vi "Open.vi"(8 "error in (no error)":errorcluster, 11 "PowerSupply-Fix in":refnum<class "PowerSupply-Fix.lvclass">) -> (0 "error out":errorcluster, 3 "PowerSupply-Fix out":refnum<class "PowerSupply-Fix.lvclass">)   [LabVIEW 2020, in "LAF2024Q2.lvlib" / "PowerSupply-Fix.lvclass"]
uses:
  PowerSupply-Fix.lvclass
  PowerSupply-Fix.lvclass/PowerSupply-Fix.ctl
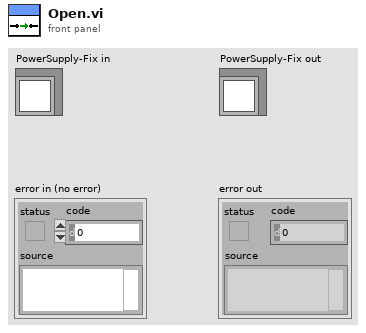
[diagram p1: front panel]
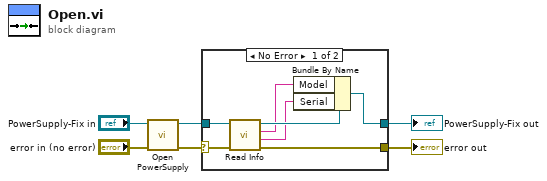
[diagram p0: block diagram]
diagram:
  n1 = call-dynamic "Open PowerSupply.vi"("error in (no error)"="error in (no error)", "PowerSupply-Fix in"="PowerSupply-Fix in") -> ("error out"=w5:errorcluster, "PowerSupply-Fix out"=w2:refnum<class "PowerSupply-Fix.lvclass">)  [unwired: 8 in]
  n2 = case shown="No Error" w5 {
    selector: w5 -> [w13 w14]
    tunnel: [w12 w14] -> w3
    tunnel: w2 -> [w11 w15]
    tunnel: [w9 w15] -> w1
    frame No Error {
      n3 = call-dynamic "Read Info.vi"("error in (no error)"=w13, "PowerSupply-Fix in"=w11) -> ("error out"=w12:errorcluster, "Serial"=w7:string, "Model"=w8:string, "PowerSupply-Fix out"=w10:refnum<class "PowerSupply-Fix.lvclass">)  [unwired: 6 in]
      n4 = Bundle By Name(cluster=w10, "Model"=w8, "Serial"=w7) -> (w9:refnum<class "PowerSupply-Fix.lvclass">)
    }
    frame Error {
    }
  }
  "error out" <- w3
  "PowerSupply-Fix out" <- w1
